vi "Identity (Read).vi"(6 "ISOBUS address":T1=-1 caption="ISOBUS address (-1)", 8 "error in":errorcluster, 11 "Mercury Reference In":T2) -> (0 "error out":errorcluster, 1 "S/W Version":string, 2 "Serial Number":string, 3 "Mercury Reference Out":T2, 4 "Instrument Valid?":bool)   [LabVIEW 2015, in "Mercury iXX.lvlib" / "System.lvlib"]
doc: "Read the identify response of the intrument."
uses:
  System.lvlib
  Controls/Mercury Reference.ctl
  Controls/Comms Transport Layer.ctl
  private/Controls/Query Dynamic Reference.ctl
  Controls/ISOBus Address.ctl
  Mercury iXX.lvlib
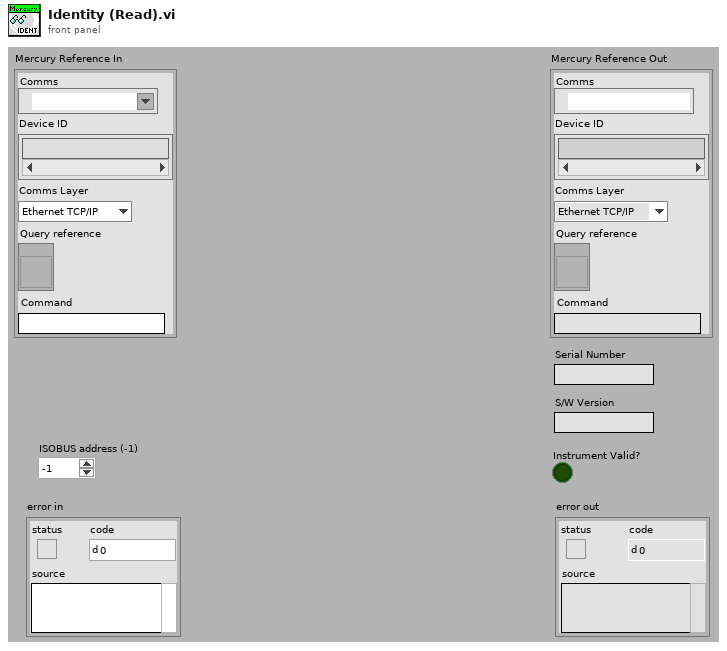
[diagram p1: front panel]
types:
  T1 = typedef "Mercury iXX.lvlib/ISOBus Address.ctl" = i32
  T2 = typedef "Mercury iXX.lvlib/Mercury Reference.ctl" = cluster{"Comms":refnum<visa-resource-name>, "Device ID":string[], "Comms Layer":T3, "Command":string, "Query reference":T4}
  T3 = typedef "Mercury iXX.lvlib/Comms Transport Layer.ctl" = enum16{"Ethernet TCP/IP", "USB", "ISOBus - RS-232", "GPIB"}
  T4 = typedef "Mercury iXX.lvlib/Query Dynamic Reference.ctl" = refnum<vi>
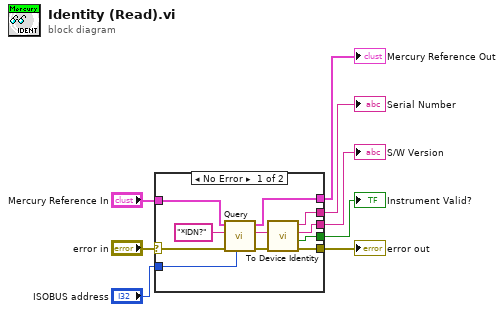
[diagram p0: block diagram]
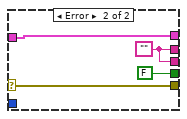
[diagram p2: hidden frame]
diagram:
  n1 = case shown="No Error" "error in" {
    selector: "error in" -> [w17 w22]
    tunnel: "Mercury Reference In" -> [w19 w23]
    tunnel: [w18 w23] -> w7
    tunnel: [w12 w22] -> w6
    tunnel: "ISOBUS address" -> [w15 _]
    tunnel: [w11 FALSE ("Valid?")] -> w3
    tunnel: [w10 w20] -> w2
    tunnel: [w9 w20] -> w1
    frame No Error {
      n2 = call "Query.vi"("ISOBUS address"=w15, "error in"=w17, "Command"="*IDN?", "Mercury Reference In"=w19) -> ("error out"=w14:errorcluster, "Data"=w13:string, "Mercury Reference Out"=w18:T2)  [unwired: 1 in, 4 out]
      n3 = call "To Device Identity.vi"("error in"=w14, "System Identifier"=w13) -> ("error out"=w12:errorcluster, "Instrument Valid"=w11:bool, "S/W Version"=w9:string, "Serial Number"=w10:string)  [unwired: 6 out]
    }
    frame Error {
      w20 = ""
    }
  }
  "Mercury Reference Out" <- w7
  "error out" <- w6
  "Instrument Valid?" <- w3
  "S/W Version" <- w1
  "Serial Number" <- w2
